vi "Test Circular Buffer.vi"() -> ()   [LabVIEW 2019]
uses:
  src/subVIs/Circular Buffer (single).vi
  src/subVIs/Circular Buffer (waveform).vi
  <vilib>/measure/NI_MABase.lvlib
  src/xy_utilities.lvlib
panel:
  in  "Boolean":bool
  out "XY Graph":cluster{"X-array":dbl[], "Y-array":dbl[]}(graph)
  out "Waveform Graph 2":waveform(dbl)(graph)
  in  "Amplitude":dbl=1.0
  in  "Frequency":dbl=11.0
  in  "signal type":T1(ring)
  in  "#S":dbl=1.0
  out "Waveform Graph":waveform(dbl)(graph)
  in  "Stop":bool
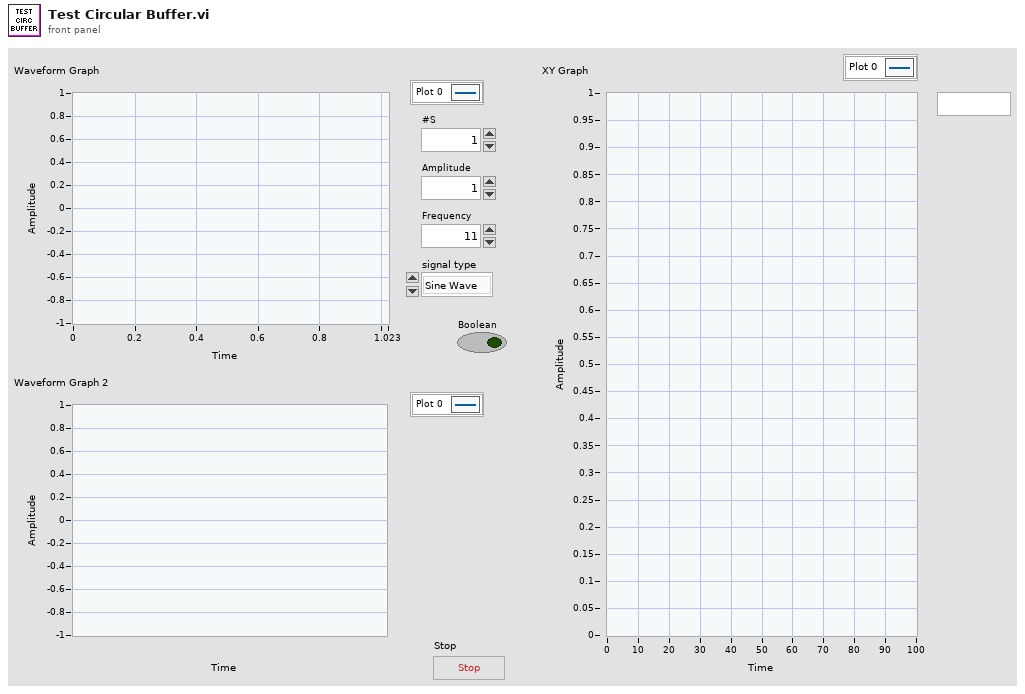
[diagram p1: front panel]
types:
  T1 = enum16{"Sine Wave", "Triangle Wave", "Square Wave", "Sawtooth Wave"}
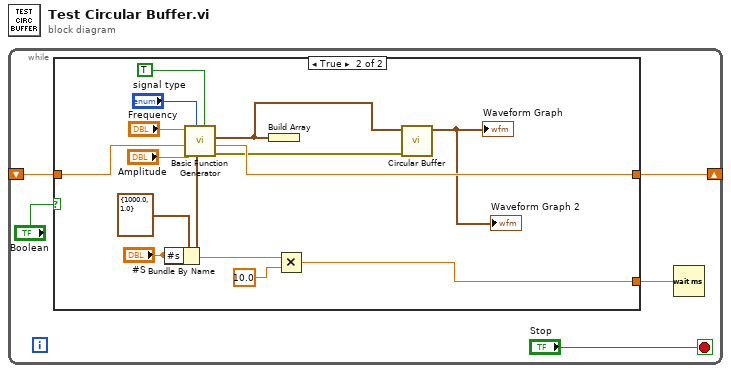
[diagram p0: block diagram]
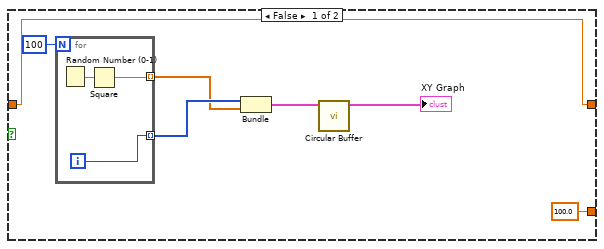
[diagram p2: hidden frame]
diagram:
  n1 = while {
    shift-right: [w4] -> _
    shift-left: _ -> [w3]
    stop <- "Stop" stop-if-true
    n2 = case shown="True" "Boolean" {
      tunnel: [w7 w25] -> w4
      tunnel: w3 -> [w7 w24]
      tunnel: [100.0 w16] -> w2
      frame False {
        n3 = for {
          N: 100 -> [_]
          tunnel: [w14] -> w10 mode=indexing
          tunnel: [w13] -> w11 mode=indexing
          i -> [w13]
          n4 = Random Number (0-1)() -> (number: 0 to 1=w15:dbl)
          n5 = Square(x=w15) -> (x^2=w14:dbl)
        }
        n6 = Bundle(w11, w10) -> (w9:cluster{i32[], dbl[]})  [unwired: 1 in]
        n7 = call-poly "Circular Buffer.vi"("XY-data"=w9) -> ("XY-data out"=→"XY Graph":cluster{"X-array":dbl[], "Y-array":dbl[]})  [unwired: 9 in, 1 out]
      }
      frame True {
        n8 = Bundle By Name(cluster=cluster{"Fs":dbl, "#s":dbl} {"Fs"=1000.0, "#s"=1.0} ("sampling info"), "#s"="#S") -> (w27:cluster{"Fs":dbl, "#s":dbl})
        n9 = call <vilib>:"Basic Function Generator.vi"("reset signal"=TRUE, "sampling info"=w27, "signal type"="signal type", "phase"=w24, "amplitude"="Amplitude", "frequency"="Frequency") -> ("error out"=w18:errorcluster, "phase out"=w25:dbl, "signal out"=w17:waveform(dbl))  [unwired: 3 in]
        n10 = Build Array(w17) -> ()  [unwired: 1 out]
        n11 = Multiply(x="#S", y=10.0) -> (x*y=w16:dbl)
        n12 = call-poly "Circular Buffer.vi"("error in"=w18, "Waveform in"=w17) -> ("Waveform out"=→"Waveform Graph" →"Waveform Graph 2":waveform(dbl))  [unwired: 8 in, 1 out]
      }
    }
    n13 = Wait (ms)(milliseconds to wait=w2) -> ()  [unwired: 1 out]
  }
